vi "Change Cursor Icon.vi"() -> ()   [LabVIEW 2023]
doc: "Demonstrates the use of the Cursor VIs to change the cursor icon while a VI is running. A picture ring is used to display all possible cursor icons. The first 6 icons in the picture ring are OS dependent. All other cursor icons in the picture ring are the same on any OS."
uses:
  <vilib>/Utility/cursorutil.llb/Set Cursor (Icon Pict).vi
  <vilib>/Utility/cursorutil.llb/Set Cursor (Cursor ID).vi
panel:
  in  "Use Previous Icon":bool
  in  "Stop":bool
  in  "Cursor Icon":u16(ring)
  # "Overview: Demonstrates the use of the Cursor VIs to programmatically manipulate the appearance of the mouse cursor.\nInstructions:\n1. Run the VI.\n2. Change the value of the Cursor Icon picture ring to change the appearance of the mouse cursor.\n3. Click the Use Previous Icon button to switch to the previous cursor icon.\n4. Click Stop to stop the VI."
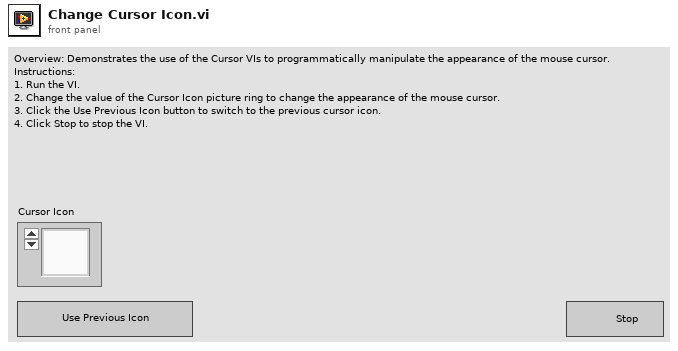
[diagram p1: front panel]
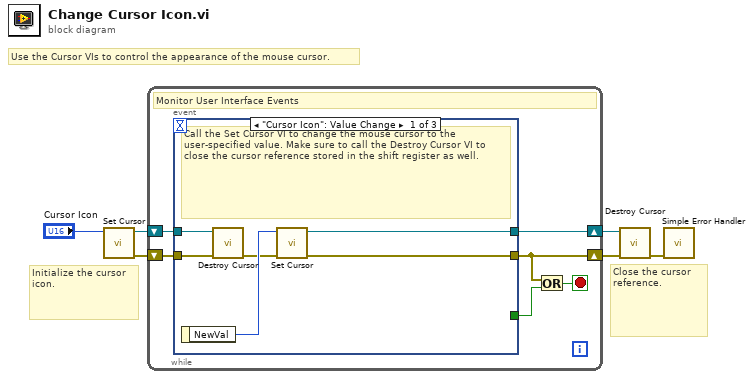
[diagram p0: block diagram]
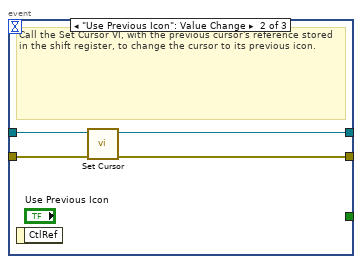
[diagram p2: hidden frame]
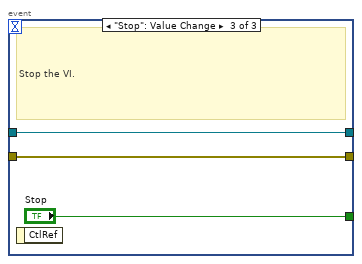
[diagram p3: hidden frame]
diagram:
  # "Use the Cursor VIs to control the appearance of the mouse cursor."
  # "Close the cursor reference."
  # "Initialize the cursor icon."
  n1 = call-poly <vilib>:"Set Cursor.vi"("icon"="Cursor Icon") -> ("error out"=w3:errorcluster, "previous cursor ID"=w2:refnum<k1>)  [unwired: 9 in]
  n2 = while {
    shift-right: [w8] -> w5
    shift-left: w3 -> [w12]
    shift-right: [w10] -> w6
    shift-left: w2 -> [w9]
    stop <- w11 stop-if-true
    # "Monitor User Interface Events"
    n3 = event shown="[0] \"Cursor Icon\": Value Change" {
      selector: _ -> [_ _ _]
      dyn-events: _ -> [_ _ _]
      timeout: _ -> [_ _ _]
      tunnel: [w18 w20 w24] -> w8
      tunnel: w12 -> [w17 w21 w24]
      tunnel: [_ _ "Stop"] -> w7
      tunnel: [w16 w22 w23] -> w10
      tunnel: w9 -> [w13 w19 w23]
      event "Cursor Icon": Value Change {
        # "Call the Set Cursor VI to change the mouse cursor to the user-specified value. Make sure to call the Destroy Cursor VI to close the cursor reference stored in the shift register as well."
        n4 = event-data() -> ("NewVal"=w15:u16)  [unwired: 1 in]
        n5 = call <vilib>:"Destroy Cursor.vi"("cursor ID"=w13, "error in (no error)"=w17) -> ("error out"=w14:errorcluster)  [unwired: 8 in]
        n6 = call-poly <vilib>:"Set Cursor.vi"("error in (no error)"=w14, "icon"=w15) -> ("error out"=w18:errorcluster, "previous cursor ID"=w16:refnum<k1>)  [unwired: 8 in]
      }
      event "Use Previous Icon": Value Change {
        # "Call the Set Cursor VI, with the previous cursor's reference stored in the shift register, to change the cursor to its previous icon."
        n7 = event-data() -> ()  [unwired: 1 in, 1 out]
        n8 = call-poly <vilib>:"Set Cursor.vi"("error in (no error)"=w21, "cursor ID"=w19) -> ("error out"=w20:errorcluster, "previous cursor ID"=w22:refnum<k1>)  [unwired: 8 in]
      }
      event "Stop": Value Change {
        # "Stop the VI."
        n9 = event-data() -> ()  [unwired: 1 in, 1 out]
      }
    }
    n10 = Or(x=w8, y=w7) -> (x .or. y?=w11:bool)
  }
  n11 = call <vilib>:"Destroy Cursor.vi"("cursor ID"=w6, "error in (no error)"=w5) -> ("error out"=w4:errorcluster)  [unwired: 8 in]
  n12 = call <vilib>:"Simple Error Handler.vi"("error in (no error)"=w4) -> ()  [unwired: 4 in, 5 out]
